vi "PrzódL.vi"(11 "Konfiguracja":T2 {"Ki" format="%.1f"; "Kp" format="%.1f"; "Prąd" format="%.1f"}) -> (3 "Message Cluster":T3)   [LabVIEW 2015]
uses:
  QMH Fundamentals - Message Cluster.ctl
  ramki konfiguracyjne.ctl
  CANFrameControl.ctl
panel:
  out "output cluster":T1 {"type" items=["CAN Data", "CAN Remote"]; "identifier" format="%.0x"}
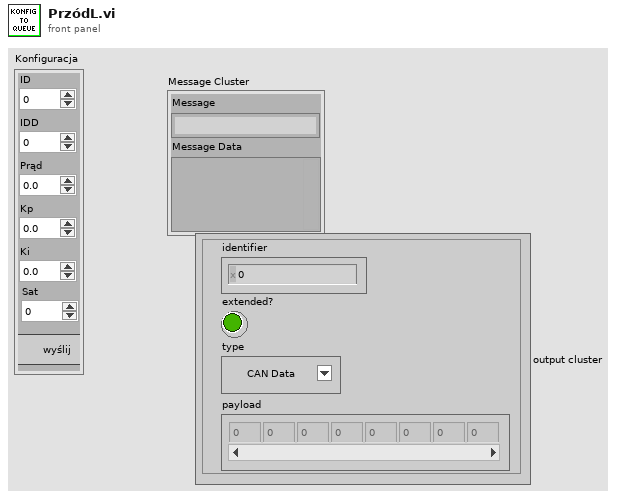
[diagram p1: front panel]
types:
  T1 = typedef "CANFrameControl.ctl" = cluster{"identifier":u32, "extended?":bool, "type":u8, "payload":u8[]}
  T2 = typedef "ramki konfiguracyjne.ctl" = cluster{"Prąd":dbl, "Kp":dbl, "Ki":dbl, "OK Button":bool, "ID":u32, "IDD":u8, "Sat":u8}
  T3 = typedef "QMH Fundamentals - Message Cluster.ctl" = cluster{"Message":string, "Message Data":variant}
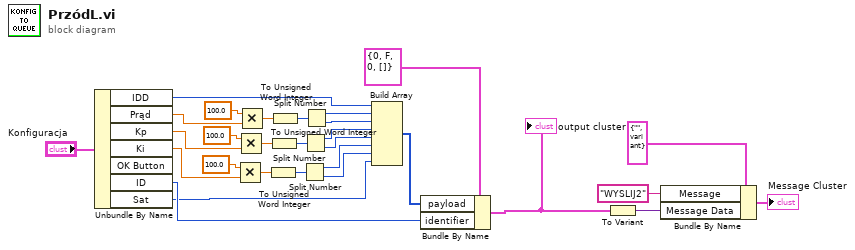
[diagram p0: block diagram]
diagram:
  n1 = Unbundle By Name("Konfiguracja") -> ("IDD"=w18:u8, "Prąd"=w17:dbl, "Kp"=w11:dbl, "Ki"=w5:dbl, "ID"=w2:u32, "Sat"=w1:u8)  [unwired: 1 out]
  n2 = Multiply(x=100.0, y=w5) -> (x*y=w6:dbl)
  n3 = Multiply(x=100.0, y=w11) -> (x*y=w12:dbl)
  n4 = Multiply(x=100.0, y=w17) -> (x*y=w20:dbl)
  n5 = To Unsigned Word Integer(number=w6) -> (unsigned 16bit integer=w8:u16)
  n6 = To Unsigned Word Integer(number=w12) -> (unsigned 16bit integer=w14:u16)
  n7 = To Unsigned Word Integer(number=w20) -> (unsigned 16bit integer=w23:u16)
  n8 = Split Number(x=w8) -> (hi(x)=w4:u8, lo(x)=w3:u8)
  n9 = Split Number(x=w14) -> (hi(x)=w10:u8, lo(x)=w9:u8)
  n10 = Split Number(x=w23) -> (hi(x)=w16:u8, lo(x)=w15:u8)
  n11 = Build Array(w18, w16, w15, w10, w9, w4, w3, w1) -> (w22:u8[])
  n12 = Bundle By Name(cluster=T1 {"identifier"=0, "extended?"=FALSE, "type"=0, "payload"=[]} ("CAN frame 2"), "payload"=w22, "identifier"=w2) -> (w29:T1)
  "output cluster" <- w29
  n13 = To Variant(anything=w29) -> (Variant=w25:variant)
  n14 = Bundle By Name(cluster=T3 {"Message"="", "Message Data"=variant} ("Message Cluster"), "Message"="WYSLIJ2", "Message Data"=w25) -> (→"Message Cluster":T3)
